vi "Open Audio File Read (Path).vi"(8 "error in (no error)":errorcluster, 11 "Path":path) -> (0 "error out":errorcluster, 3 "Audio File Refnum":T1)   [LabVIEW 2020, in "G-Audio.lvlib"]
doc: "Opens an audio file and initializes the relevant decoder.\n\nSupported codecs: flac, mp3, vorbis (ogg), and wav."
uses:
  G-Audio.lvlib
  Controls/Audio File Refnum.ctl
  Private/Result To Error.vi
  <vilib>/Utility/error.llb/Error Cluster From Error Code.vi
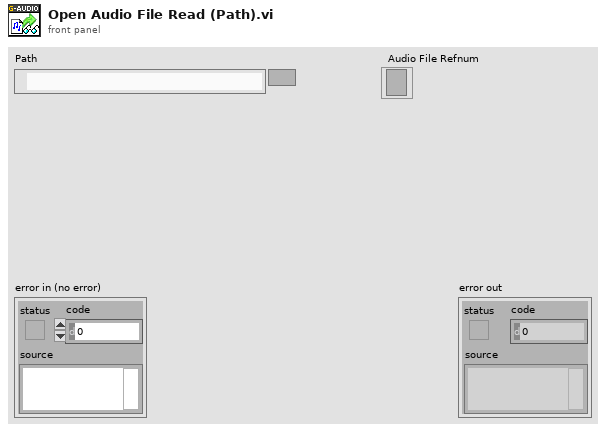
[diagram p1: front panel]
types:
  T1 = typedef "G-Audio.lvlib/Audio File Refnum.ctl" = refnum<file>
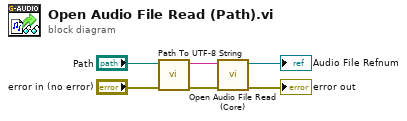
[diagram p0: block diagram]
diagram:
  n1 = call "Path To UTF-8 String.vi"("error in"="error in (no error)", "Path"="Path") -> ("error out"=w1:errorcluster, "UTF-8 String"=w5:string)  [unwired: 8 in]
  n2 = call "Open Audio File Read (Core).vi"("error in (no error)"=w1, "Path"=w5) -> ("error out"=→"error out":errorcluster, "Audio File Refnum"=→"Audio File Refnum":T1)  [unwired: 8 in]
